vi "Close.vi"(8 "error in":errorcluster, 11 "Voltage Control in":refnum<class "Voltage Control.lvclass">) -> (0 "error out":errorcluster, 3 "Voltage Control out":refnum<class "Voltage Control.lvclass">)   [LabVIEW 2023, in "Voltage Control.lvclass"]
uses:
  Voltage Control.lvclass
  Voltage Control.lvclass/Voltage Control.ctl
  <vilib>/ADAS Replay HIL/AdasHilServices/AdasHilServices Fill In Error Info Ex.vi
  <vilib>/ADAS Replay HIL/AdasHilServices/AdasHilChannelServices.lvlib
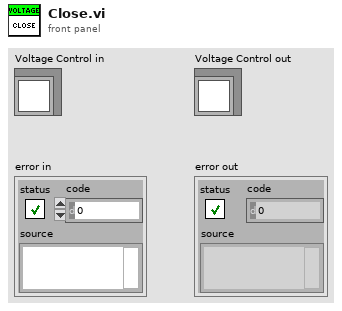
[diagram p1: front panel]
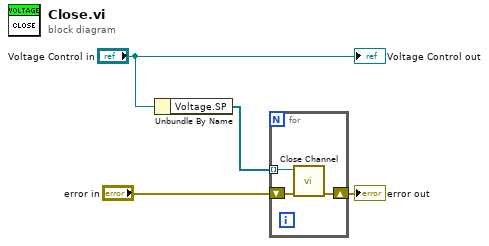
[diagram p0: block diagram]
diagram:
  n1 = Unbundle By Name("Voltage Control in") -> ("Voltage.SP"=w2:refnum<k21>[])
  n2 = for {
    tunnel: w2 -> [w5] mode=indexing
    shift-right: [w7] -> w4
    shift-left: "error in" -> [w6]
    n3 = call <vilib>:"Close Channel.vi"("error in"=w6, "ADAS HIL Channel"=w5) -> ("error out"=w7:errorcluster)  [unwired: 9 in]
  }
  "error out" <- w4
  "Voltage Control out" <- "Voltage Control in"
